vi "AddCORSHeaders.vi"(11 "Web Request in":refnum<class "Web Request.lvclass">) -> (3 "Web Request out":refnum<class "Web Request.lvclass">)   [LabVIEW 2017]
uses:
  <vilib>/wsapi/Web Request.lvclass
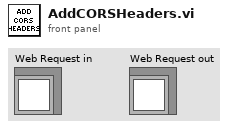
[diagram p1: front panel]
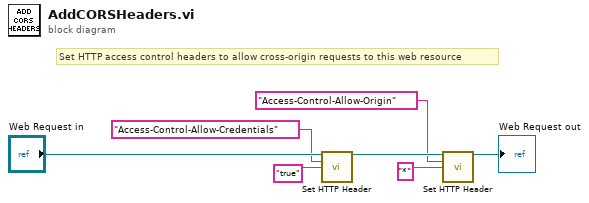
[diagram p0: block diagram]
diagram:
  # "Set HTTP access control headers to allow cross-origin requests to this web resource"
  n1 = call <vilib>:"Set HTTP Header.vi"("LabVIEW Web Service Request"="Web Request in", "header"="Access-Control-Allow-Credentials", "header value"="true") -> ("LabVIEW Web Service Request out"=w3:refnum<class "Web Request.lvclass">)  [unwired: 11 in, 1 out]
  n2 = call <vilib>:"Set HTTP Header.vi"("LabVIEW Web Service Request"=w3, "header"="Access-Control-Allow-Origin", "header value"="*") -> ("LabVIEW Web Service Request out"=→"Web Request out":refnum<class "Web Request.lvclass">)  [unwired: 11 in, 1 out]
